vi "Write gplugin for migrator.vi"(0 "Config":T1, 5 "Path":path=path "D:/EXP/ABC/ABC.gplugindata", 11 "error in (no error)":errorcluster) -> (15 "error out":errorcluster)   [LabVIEW 2021, in "G Plugin Editor.lvlib"]
uses:
  G Plugin Editor.lvlib
  controls/Data Holder.ctl
  <vilib>/xml/Load XML String.vi
  <vilib>/xml/Close Reference(Node).vi
  <vilib>/xml/NI_XML.lvlib
  <resource>/objmgr/DOMUserDefRef.rc
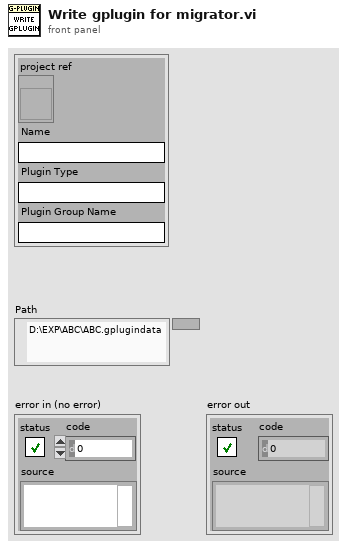
[diagram p1: front panel]
types:
  T1 = typedef "G Plugin Editor.lvlib/Data Holder.ctl" = cluster{"project ref":refnum<vi>, "Name":string, "Plugin Type":string, "Plugin Group Name":string}
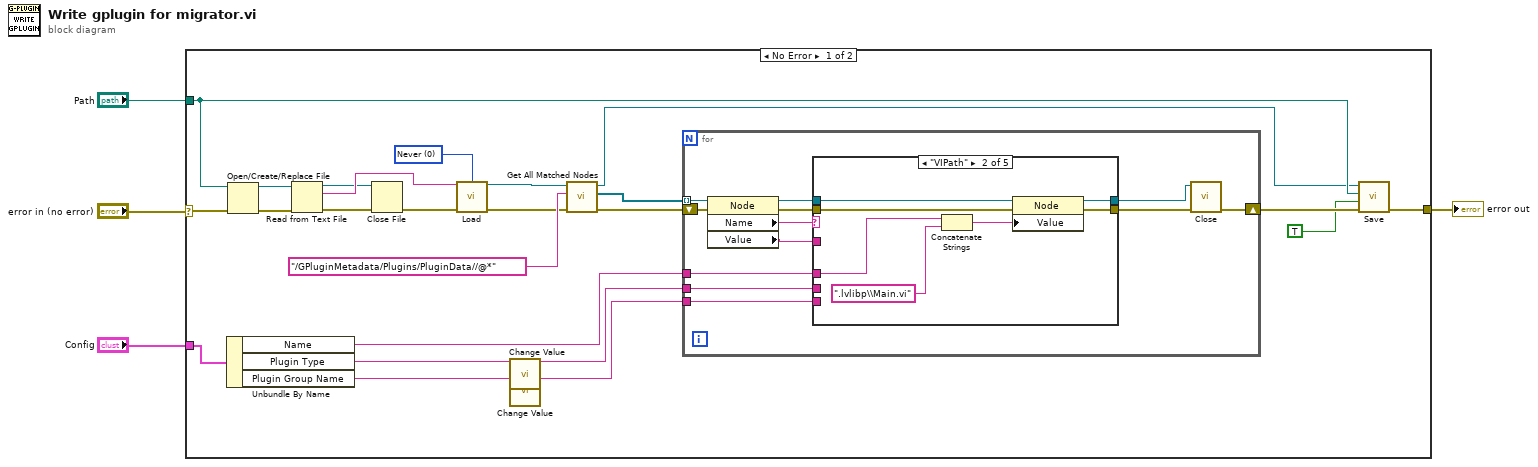
[diagram p0: block diagram]
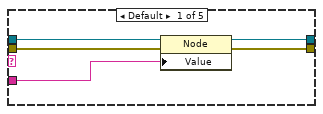
[diagram p2: hidden frame]
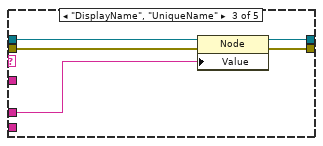
[diagram p3: hidden frame]
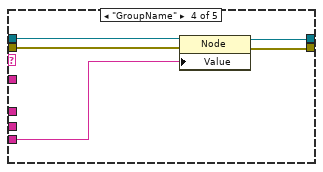
[diagram p4: hidden frame]
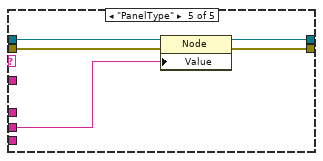
[diagram p5: hidden frame]
diagram:
  n1 = case shown="No Error" "error in (no error)" {
    selector: "error in (no error)" -> [w27 w68]
    tunnel: [w11 w68] -> w4
    tunnel: "Path" -> [w20 _]
    tunnel: "Config" -> [w10 _]
    frame No Error {
      w24 = 0 items=["Never", "Always", "Auto"] ("validate on load (Auto)")
      n2 = Unbundle By Name(w10) -> ("Name"=w9:string, "Plugin Type"=w8:string, "Plugin Group Name"=w6:string)
      n3 = Open/Create/Replace File(file path (use dialog)=w20, error in=w27) -> (refnum out=w28:refnum<file>, error out=w25:errorcluster)  [unwired: 4 in, 1 out]
      n4 = Read from Text File(file (use dialog)=w28, error in=w25) -> (refnum out=w17:refnum<file>, text=w26:string, error out=w15:errorcluster)  [unwired: 2 in, 1 out]
      n5 = Close File(refnum=w17, error in=w15) -> (error out=w16:errorcluster)  [unwired: 1 out]
      n6 = call-poly <vilib>:"Load.vi"("XML string"=w26, "validate on load (Auto)"=w24, "error in (no error)"=w16) -> ("DOM document out"=w23:refnum<k20>, "error out"=w13:errorcluster)  [unwired: 10 in, 1 out]
      n7 = call "Change Value.vi"("String"=w8) -> ("String Out"=w7:string)  [unwired: 14 in]
      n8 = call "Change Value.vi"("String"=w6) -> ("String Out"=w5:string)  [unwired: 14 in]
      n9 = call <vilib>:"Get All Matched Nodes.vi"("error in (no error)"=w13, "XPath expression"="/GPluginMetadata/Plugins/PluginData//@*", "node in"=w23) -> ("error out"=w12:errorcluster, "node result array"=w22:refnum<k20>[], "node out"=w14:refnum<k20>)  [unwired: 6 in]
      n10 = for {
        tunnel: w22 -> [w40] mode=indexing
        shift-right: [w35] -> w19
        shift-left: w12 -> [w38]
        tunnel: w9 -> [w32]
        tunnel: w7 -> [w31]
        tunnel: w5 -> [w30]
        n11 = property class="Node"(reference=w40, error in=w38) -> (reference out=w39:refnum<k20>, error out=w37:errorcluster, "Name"=w33:string, "Value"=w29:string)
        n12 = case shown="\"VIPath\"" w33 {
          tunnel: w39 -> [w45 w52 w57 w61 w67]
          tunnel: w37 -> [w42 w49 w56 w62 w65]
          tunnel: [w44 w51 w55 w59 w66] -> w36
          tunnel: [w43 w50 w54 w60 w64] -> w34
          tunnel: w32 -> [_ w48 w53 _ _]
          tunnel: w31 -> [_ _ _ _ w63]
          tunnel: w30 -> [_ _ _ w58 _]
          tunnel: w29 -> [w41 _ _ _ _]
          frame Default {
            n13 = property class="Node"(reference=w45, error in=w42, "Value"=w41) -> (reference out=w44:refnum<k20>, error out=w43:errorcluster)
          }
          frame "VIPath" {
            n14 = Concatenate Strings(w48, ".lvlibp\\Main.vi" ("string")) -> (w47:string)
            n15 = property class="Node"(reference=w52, error in=w49, "Value"=w47) -> (reference out=w51:refnum<k20>, error out=w50:errorcluster)
          }
          frame "DisplayName", "UniqueName" {
            n16 = property class="Node"(reference=w57, error in=w56, "Value"=w53) -> (reference out=w55:refnum<k20>, error out=w54:errorcluster)
          }
          frame "GroupName" {
            n17 = property class="Node"(reference=w61, error in=w62, "Value"=w58) -> (reference out=w59:refnum<k20>, error out=w60:errorcluster)
          }
          frame "PanelType" {
            n18 = property class="Node"(reference=w67, error in=w65, "Value"=w63) -> (reference out=w66:refnum<k20>, error out=w64:errorcluster)
          }
        }
        n19 = call-poly <vilib>:"Close.vi"("error in (no error)"=w34, "node"=w36) -> ("error out"=w35:errorcluster)  [unwired: 7 in]
      }
      n20 = call <vilib>:"Save.vi"("error in (no error)"=w19, "overwrite file (True)"=TRUE, "XML file path"=w20, "DOM document in"=w14) -> ("error out"=w11:errorcluster)  [unwired: 5 in, 2 out]
    }
    frame Error {
    }
  }
  "error out" <- w4
